vi "Write to CSV Test.vi"(8 "Error In":errorcluster) -> (0 "Error Out":errorcluster)   [LabVIEW 2023, in "Test.lvlib"]
doc: "The VI is a test file that checks the logging data into csv file operation using different test cases."
uses:
  Test.lvlib
  Controls/Test Input.ctl
  <vilib>/Utility/file.llb/Read Delimited Spreadsheet (string).vi
  <vilib>/addons/_JKI Toolkits/Caraya/classes/Assert/Assert Equal Value_Variant.vi
  <vilib>/addons/_JKI Toolkits/Caraya/classes/Assert/Assert.lvclass
  <vilib>/addons/_JKI Toolkits/Caraya/classes/Test/Test.lvclass
  File Path Operations/File and Path Operations.lvlib
panel:
  # "WRITE TO CSV TEST"
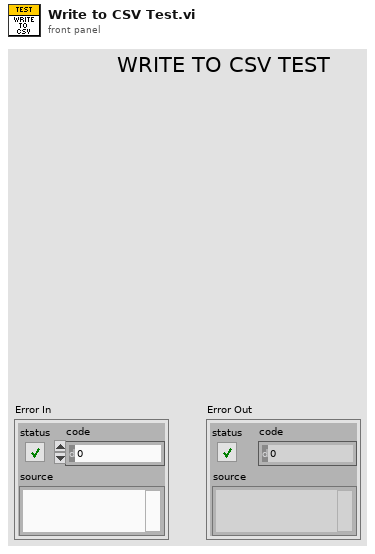
[diagram p1: front panel]
types:
  T1 = typedef "Test.lvlib/Test Input.ctl" = cluster{"Test Input":string[][]}
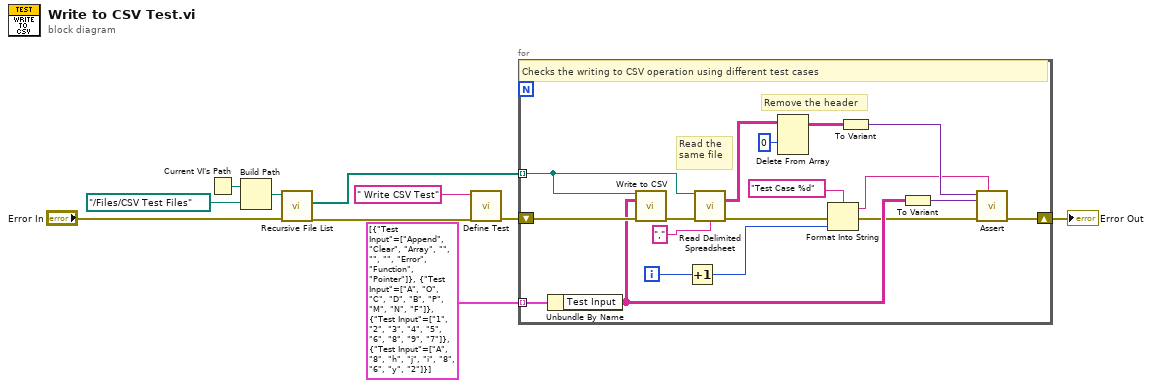
[diagram p0: block diagram]
diagram:
  n1 = Current VI's Path() -> (path=w4:path)
  n2 = Build Path(base path=w4, name or relative path=path "../Files/CSV Test Files") -> (appended path=w7:path)
  n3 = call <vilib>:"Recursive File List.vi"("error in (no error)"="Error In", "Folder Path"=w7) -> ("error out"=w6:errorcluster, "All Files in Dir"=w5:path[])  [unwired: 5 in, 3 out]
  n4 = call <vilib>:"Define Test.vi"("error in (no error)"=w6, "Label (VI Title)"=" Write CSV Test") -> ("error out"=w9:errorcluster)  [unwired: 8 in, 1 out]
  n5 = for {
    tunnel: w5 -> [w19] mode=indexing
    shift-right: [w26] -> w3
    shift-left: w9 -> [w25]
    tunnel: T1[] [{"Test Input"=[["Append", "Clear", "Array"], ["", "", ""], ["Error", "Function", "Pointer"]]}, {"Test Input"=[["A", "O", "C"], ["D", "B", "P"], ["M", "N", "F"]]}, {"Test Input"=[["1", "2", "3"], ["4", "5", "6"], ["8", "9", "7"]]}, {"Test Input"=[["A", "8", "h"], ["j", "i", "8"], ["6", "y", "2"]]}] -> [w24] mode=indexing
    i -> [w28]
    # "Remove the header"
    # "Read the same file"
    # "Checks the writing to CSV operation using different test cases"
    n6 = Unbundle By Name(w24) -> ("Test Input"=w21:string[][])
    n7 = call "Write to CSV.vi"("Path In"=w19, "Array In"=w21, "Error In"=w25) -> ("Error Out"=w13:errorcluster)  [unwired: 10 in, 2 out]
    n8 = Increment(x=w28) -> (x+1=w27:i32)
    n9 = call-poly <vilib>:"Read Delimited Spreadsheet.vi"("file path (dialog if empty)"=w19, "error in (no error)"=w13, "delimiter (\\t)"="," ("delimiter (\\t)")) -> ("all rows"=w16:string[][], "error out"=w14:errorcluster)  [unwired: 7 in, 4 out]
    n10 = Delete From Array(array=w16, index (row)=0) -> (array with subset deleted=w15:string[][])  [unwired: 2 in, 1 out]
    n11 = Format Into String(format string="Test Case %d", error in=w14, w27) -> (resulting string=w11:string, error out=w20:errorcluster)  [unwired: 1 in]
    n12 = To Variant(anything=w15) -> (Variant=w22:variant)
    n13 = To Variant(anything=w21) -> (Variant=w23:variant)
    n14 = call-poly <vilib>:"Assert.vi"("Label"=w11, "error in (no error)"=w20, "Y"=w23, "X"=w22) -> ("error out"=w26:errorcluster)  [unwired: 6 in, 1 out]
  }
  "Error Out" <- w3
